vi "waitOnIRQ.vi"(8 "error in (no error)":errorcluster, 10 "Timeout (ms)":i32, 11 "Modbus in":refnum<class "Modbus.lvclass">) -> (0 "error out":errorcluster, 1 "TimedOut":bool, 2 "IRQs":i32[](array[numeric]), 3 "Modbus out":refnum<class "Modbus.lvclass">)   [LabVIEW 2016, in "RTModbusFPGA.lvlib" / "Modbus.lvclass"]
uses:
  Modbus.lvclass
  Modbus.lvclass/Modbus.ctl
  Common_RT_FPGA/IIRQ/IIRQ.lvclass
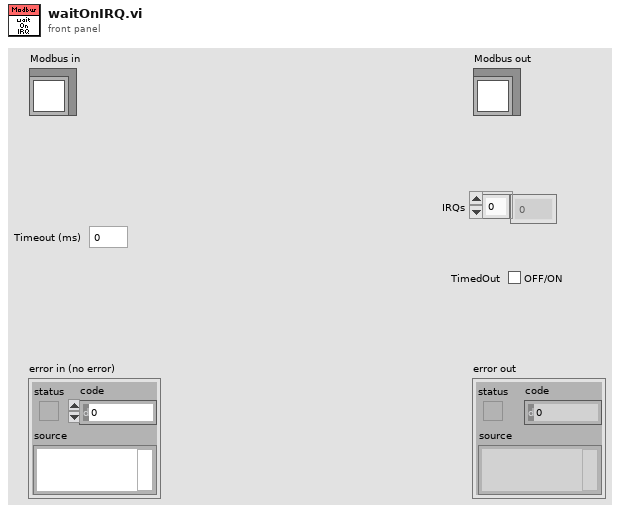
[diagram p1: front panel]
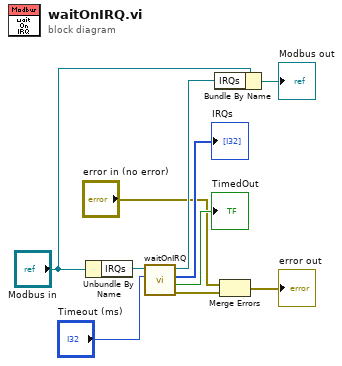
[diagram p0: block diagram]
diagram:
  n1 = Unbundle By Name("Modbus in") -> ("IRQs"=w10:refnum<class "IIRQ.lvclass">)
  n2 = call-dynamic "waitOnIRQ.vi"("Timeout"="Timeout (ms)", "IIRQ in"=w10) -> ("error out"=w3:errorcluster, "TimedOut"=→"TimedOut":bool, "IRQs"=→"IRQs":i32[], "IIRQ out"=w7:refnum<class "IIRQ.lvclass">)  [unwired: 6 in]
  n3 = Bundle By Name(cluster="Modbus in", "IRQs"=w7) -> (→"Modbus out":refnum<class "Modbus.lvclass">)
  n4 = Merge Errors("error in (no error)", w3) -> (→"error out":errorcluster)
